vi "3_Speech_Rec_Deploy(file).vi"() -> ()   [LabVIEW 2020]
doc: "This example demonstrates the usage of Deep Learning Toolkit for loading the model pretrained for speech recognition and running for inference."
uses:
  <vilib>/Ngene/Deep Learning Toolkit/Toolkit/NN_Network/Controls/NN_Device.ctl
  <vilib>/Ngene/Deep Learning Toolkit/Toolkit/NN_Network/Controls/NN_Save_Before_Destroy_Options.ctl
  <vilib>/Ngene/Deep Learning Toolkit/Toolkit/NN_Network/API/NN_Set_Input/3D/NN_Set_Input(3D_SGL_idx).vi
  <vilib>/Ngene/Deep Learning Toolkit/Toolkit/Deep_Learning_Toolkit_by_Ngene.lvlib
  <vilib>/vision/NI_Vision_Development_Module.lvlib
panel:
  out "Spectrogram":dbl[][](graph)
  out "Class Labels":string[](array[string])=["dog", "down", "go", "forward", "four", "stop", "backward", "bed", "bird", "learn", "off", "five", "follow", "one", "no", "seven", "on", "cat", "wow", "_background_noise_", "nine", "left", "marvin", "zero", "up", "right", "sheila", "yes", "visual", "six", "two", "house", "eight", "tree", "happy", "three"]
  out "Waveform":waveform(dbl)(graph)={"t0"=timestamp(0 s since 1904-01-01), "dt"=6.25e-05, "Y"=array[16000 elements]}
  out "Class Probabilities":sgl[](array[slide])=[0.99914944, 0.0004657383, 9.833006e-05, 9.4494404e-05, 6.293928e-05, 5.5525186e-05, 1.9071045e-05, 1.3614067e-05, 8.803039e-06, 7.138225e-06, 4.5331067e-06, 4.472217e-06, 3.2921575e-06, 2.4475762e-06, 2.2857214e-06, 2.1201042e-06, 1.2650248e-06, 1.2449445e-06, 1.0311046e-06, 5.384098e-07, 3.8239716e-07, 2.570093e-07, 2.0991196e-07, 1.9032325e-07, 1.7803737e-07, 1.6300649e-07, 1.211693e-07, 9.199508e-08, 4.1726615e-08, 1.04164135e-08, 9.058018e-09, 5.2775126e-09, 2.9758322e-09, 2.9543528e-09, 1.9944413e-09, 8.306618e-10] scale=0.0..1.0
  in  "NN Device":T1=enum."GPU"
  in  "Path to wav":path=path "C:/Users/Nahapet/Downloads/data_speech_commands_v0.02/dog/0ac15fe9_nohash_2.wav"
  in  "Play?":bool=TRUE
  out "Inference Time(sec)":dbl=0.07463920000009239 format="%#_3p"
  in  "Network Configuration File Path":path=path "D:/working/speech_rec/Speech_Rec_net_cfg_26_07_10__17_58_19.cfg"
  in  "Weight File Path":path=path "D:/working/speech_rec/Speech_Rec_weights_26_07_10__17_58_19.bin"
  in  "Stop":bool
  # "Overview: This example demonstrates the use of Deep Learning Toolkit for loading a model pretrained for speech recognition and running it for inference.\nRequirements:\n1. Deep Learning Toolkit for LabVIEW.\n2. NI Vision Development Module.\nInstructions:\nThis example requires the trained model (network topology file .cfg and trained weights file .bin) generated in the previous step.\n1. Provide the trained model files at \"Network Configuration File Path\" and \"Weight File Path\".\n2. Run the VI.\n3. Drag and drop a wav file into the \"Path to wav\" control and observe the prediction results."
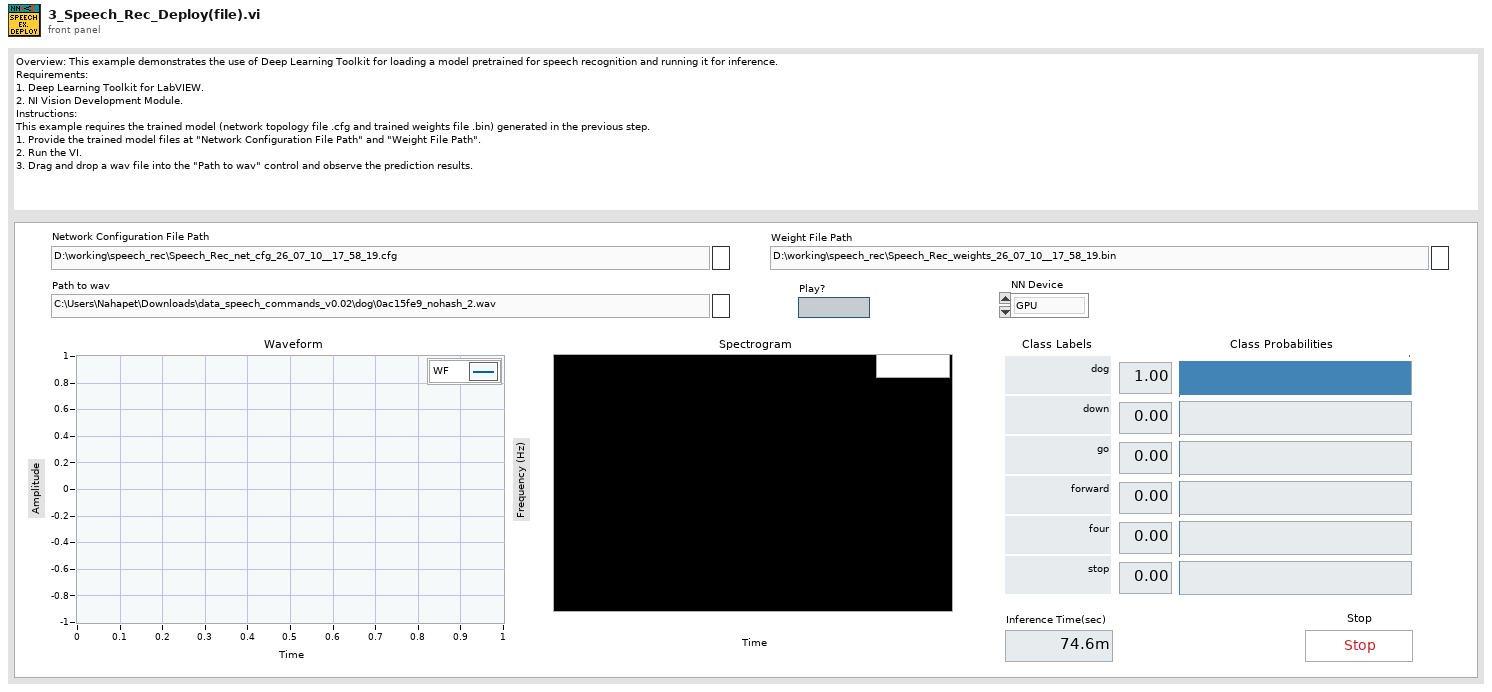
[diagram p1: front panel]
types:
  T1 = typedef "Deep_Learning_Toolkit_by_Ngene.lvlib/NN_Device.ctl" = enum16{"CPU", "GPU"}
  T2 = typedef "Image Type" = u32
  T3 = typedef "Deep_Learning_Toolkit_by_Ngene.lvlib/NN_Save_Before_Destroy_Options.ctl" = cluster{"CFG?":bool, "Weights?":bool, "Render?":bool}
  T4 = typedef "Deep_Learning_Toolkit_by_Ngene.lvlib/NN_Config_Params.ctl" = cluster{"Name":string, "mBatch":i32, "NN_Train_Params":T5, "LR_Decay_Policy":T8, "Labels":string[], "Loss":T10, "Max_WS_Size(B)":i64, "DryRun?":bool}
  T5 = typedef "Deep_Learning_Toolkit_by_Ngene.lvlib/NN_Train_Params.ctl" = cluster{"Optimizer":T6, "Beta_1":sgl, "Beta_2":sgl, "Weight Decay(L1)":sgl, "Weight Decay(L2)":sgl, "Data_Sampling":T7}
  T6 = typedef "Deep_Learning_Toolkit_by_Ngene.lvlib/NN_Train_Optimizer.ctl" = enum16{"SGD", "Adam", "Adagrad", "Adadelta", "RMSProp", "Nesterov"}
  T7 = typedef "Deep_Learning_Toolkit_by_Ngene.lvlib/NN_Train_Data_Sampling.ctl" = enum16{"Random", "Sequential"}
  T8 = typedef "Deep_Learning_Toolkit_by_Ngene.lvlib/NN_LR_Policy_Cfg.ctl" = cluster{"Policy_Type":T9, "LR0":dbl, "k":sgl, "WarmUp_Policy":enum16{"Step", "Ramp"}, "WarmUp_Iter":i32, "WarmUp_Ratio":sgl}
  T9 = typedef "Deep_Learning_Toolkit_by_Ngene.lvlib/NN_LR_Policy_Type.ctl" = enum16{"Manual", "Step", "Exp", "1/t"}
  T10 = typedef "Deep_Learning_Toolkit_by_Ngene.lvlib/NN_Loss_Config_Params.ctl" = cluster{"Loss_Type":T11, "Loss_Conf_Params":variant}
  T11 = typedef "Deep_Learning_Toolkit_by_Ngene.lvlib/NN_Loss_Type.ctl" = enum16{"None", "MSE", "CrossEntropy", "YOLO_v2", "YOLO_v4"}
  T12 = typedef "Deep_Learning_Toolkit_by_Ngene.lvlib/NN_Layer_Config_Params.ctl" = cluster{"Layer_Type":T13, "Layer_Conf_Params":variant, "Input Layers":string[]}
  T13 = typedef "Deep_Learning_Toolkit_by_Ngene.lvlib/NN_Layer_Type.ctl" = enum16{"Input1D", "Input3D", "Conv1D", "Conv2D", "Conv2D_Adv", "MaxPool", "AvgPool", "UpSample", "DropOut3D", "ShortCut", "Concat", "SoftMax3D", "FC", "DropOut", "Softmax", "Flatten", "YOLO_v2", "YOLO_v4", "Activation", "BatchNormalization", "LayerNormalization", "Scale", "Unsupported"}
  T14 = typedef "Deep_Learning_Toolkit_by_Ngene.lvlib/NN.ctl" = cluster{"Name":string, "No of Layers":i32, "mBatch":i32, "Layers":T15[], "Dimty":T16, "Dims_In":T17, "Dims_Out":T17, "Working_Dir":path, "Train?":bool, "Train_Params":T5, "LR_Update_Policy":T8, "Session Data":T18, "Ground_truth":T19, "NNg_hdls":T20, "NN_Device":T1, "GPU Id":i32, "Labels":string[], "Loss_Type":T11, "Loss_Cfg_Prms":variant, "NNG_WS":T21, "DryRun?":bool}
  T15 = typedef "Deep_Learning_Toolkit_by_Ngene.lvlib/NN_Layer_ref.ctl" = refnum<file>
  T16 = typedef "Deep_Learning_Toolkit_by_Ngene.lvlib/NN_In_Out_Dim-ty.ctl" = enum8{"In1D_Out1D", "In3D_Out1D", "In3D_Out3D", "In3D_OutBBox"}
  T17 = typedef "Deep_Learning_Toolkit_by_Ngene.lvlib/NN_Dims(C,H,W).ctl" = cluster{"C":i32, "H":i32, "W":i32}
  T18 = typedef "Deep_Learning_Toolkit_by_Ngene.lvlib/NN_Train_Session_Data.ctl" = cluster{"Epochs":sgl, "Tot_Iter":i32, "LR":sgl, "LR_iter":i32}
  T19 = typedef "Deep_Learning_Toolkit_by_Ngene.lvlib/NN_Ground_truth.ctl" = cluster{"Y":variant}
  T20 = typedef "Deep_Learning_Toolkit_by_Ngene.lvlib/nng_cuda_handles.ctl" = cluster{"cudnn":u64, "cublas":u64, "stream":u64, "curand":u64}
  T21 = typedef "Deep_Learning_Toolkit_by_Ngene.lvlib/NNG_WS.ctl" = cluster{"NNG_WS_Mem":T22, "Max_WS_Size":i64}
  T22 = typedef "Deep_Learning_Toolkit_by_Ngene.lvlib/NNg_WS_Mem_DVR.ctl" = refnum<data-value>
  T23 = typedef "IMAQ Image.ctl" = refnum<image>
  T24 = cluster{"spectral map":dbl[][], "X scale":cluster{"offset":dbl, "multiplier":dbl}, "Y scale":cluster{"offset":dbl, "multiplier":dbl}, "attribute":variant}
  T25 = typedef "Deep_Learning_Toolkit_by_Ngene.lvlib/NN_Layer.ctl" = cluster{"Name":string, "Layer_Data":T26, "Layer_Type":T13, "Dims_In":T17, "Layers_In":T15[], "Dims_Out":T17, "Layers_Out":T15[], "Metrics":T27, "GPU_Data":T28, "mBatch":i32, "NN_Device":T1, "NNg_hdls":T20, "Train?":bool, "Dimty":T29, "RecptField":T30, "Idx":i32}
  T26 = typedef "Deep_Learning_Toolkit_by_Ngene.lvlib/NN_Layer_Data_Refnum.ctl" = refnum<file>
  T27 = typedef "Deep_Learning_Toolkit_by_Ngene.lvlib/NN_Layer_Metrics.ctl" = cluster{"Data":dbl, "Params":dbl, "Ops":dbl}
  T28 = typedef "Deep_Learning_Toolkit_by_Ngene.lvlib/NNg_Layer_Data_Refnum.ctl" = refnum<file>
  T29 = typedef "Deep_Learning_Toolkit_by_Ngene.lvlib/NN_Layer_Dimty.ctl" = enum16{"1D", "3D"}
  T30 = typedef "Deep_Learning_Toolkit_by_Ngene.lvlib/NN_Layer_RF_State.ctl" = cluster{"Dims":T31, "J":T31}
  T31 = typedef "Deep_Learning_Toolkit_by_Ngene.lvlib/NN_Dims(V,H).ctl" = cluster{"V":i32, "H":i32}
  T32 = cluster{"Numeric Control":sgl, "Labels":string}[]
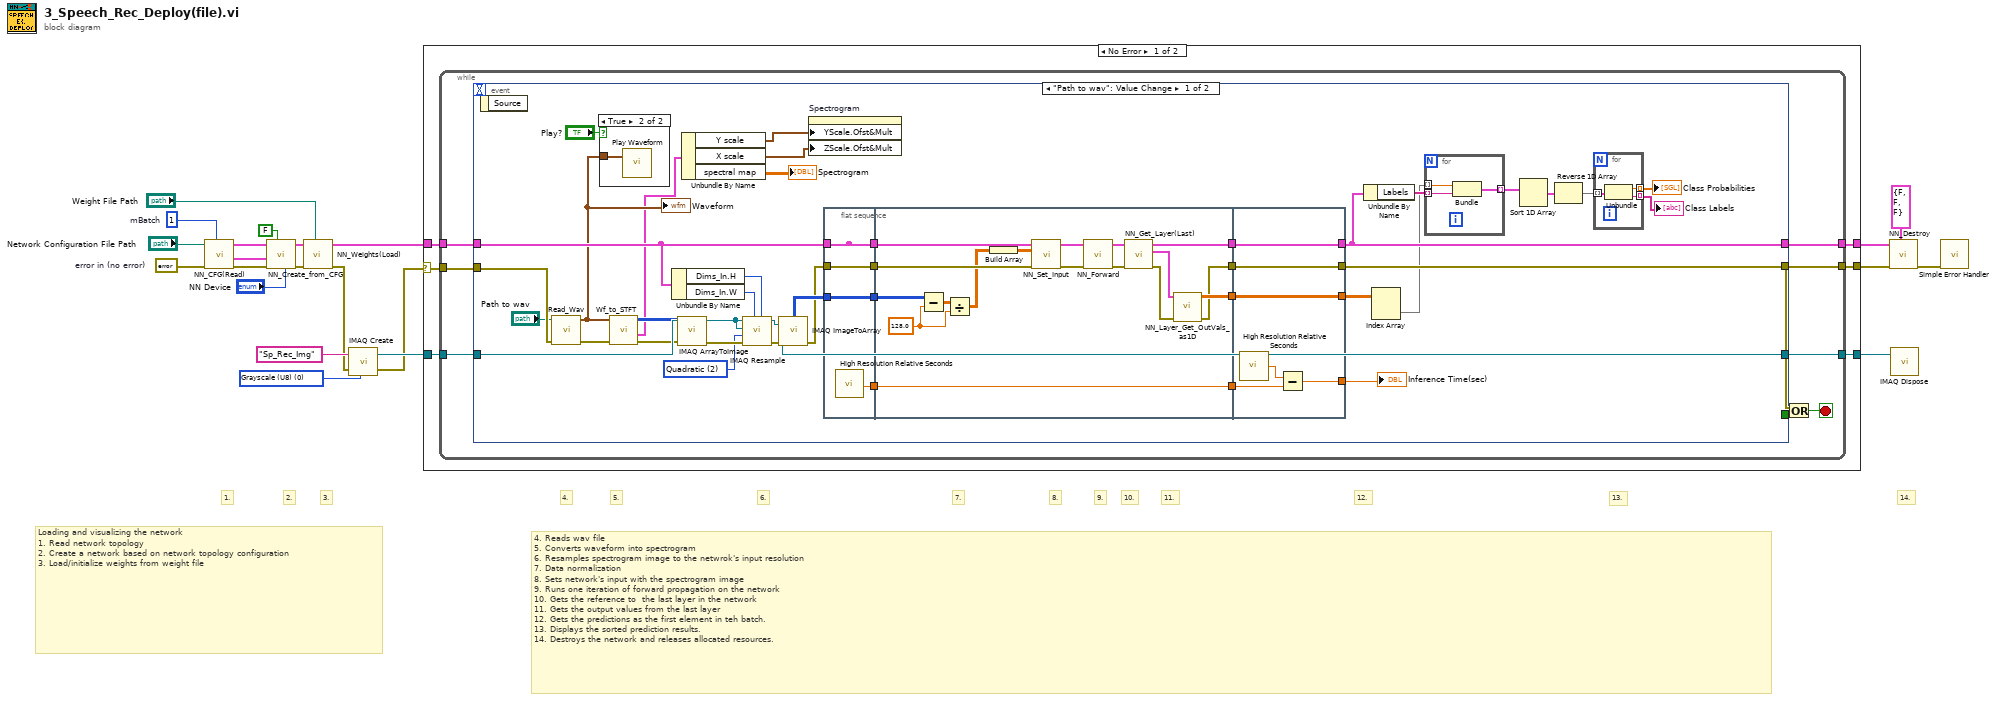
[diagram p0: block diagram]
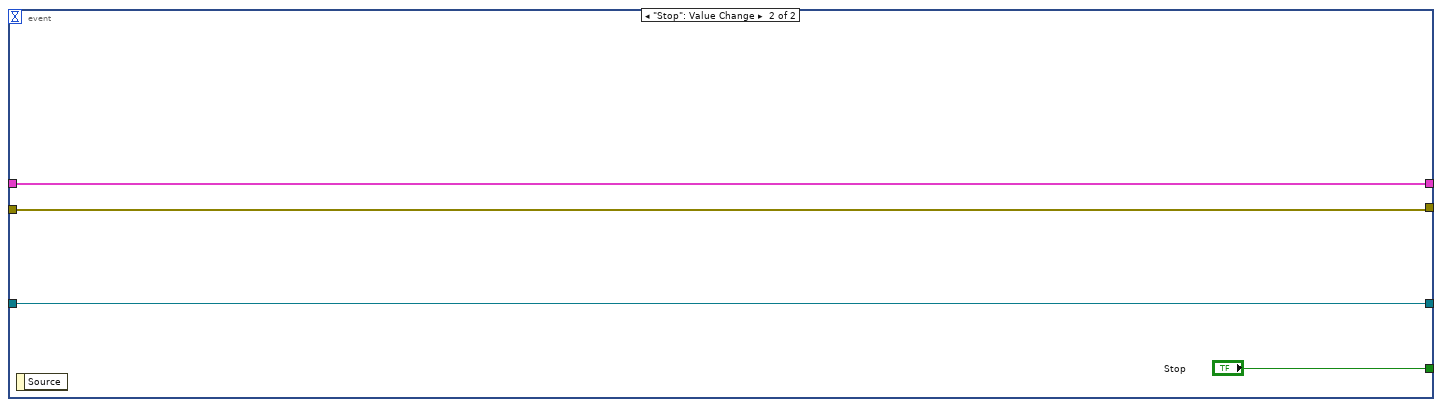
[diagram p3: hidden frame]
diagram:
  w2 = 1  # mBatch
  w14 = errorcluster {"status"=FALSE, "code"=0, "source"=""}  # error in (no error)
  w18 = T2 0 items=["Grayscale (U8)", "Grayscale (I16)", "Grayscale (SGL)", "Complex (CSG)", "RGB (U32)", "HSL (U32)", "RGB (U64)", "Grayscale (U16)"] ("Image Type")
  # "13."
  # "14."
  # "12."
  # "11."
  # "10."
  # "9."
  # "4. Reads wav file\n5. Converts waveform into spectrogram\n6. Resamples spectrogram image to the netwrok's input resolution\n7. Data normalization\n8. Sets network's input with the spectrogram image\n9. Runs one iteration of forward propagation on the network\n10. Gets the reference to  the last layer in the network\n11. Gets the output values from the last layer\n12. Gets the predictions as the first element in teh batch.\n13. Displays the sorted prediction results.\n14. Destroys the network and releases allocated resources."
  # "8."
  # "7."
  # "6."
  # "5."
  # "4."
  # "Loading and visualizing the network\n1. Read network topology\n2. Create a network based on network topology configuration\n3. Load/initialize weights from weight file"
  # "3."
  # "2."
  # "1."
  n1 = call <vilib>:"NN_CFG(Read).vi"("mBatch"=w2, "error in (no error)"=w14, "CFG file path"="Network Configuration File Path") -> ("error out"=w16:errorcluster, "Net_Cfg"=w15:T4, "Layer_Cfg"=w6:T12[])  [unwired: 6 in]
  n2 = call <vilib>:"NN_Create_from_CFG.vi"("NN_Device"="NN Device", "Train? (false)"=FALSE, "error in (no error)"=w16, "Net_Cfg"=w15, "Layer_Cfg"=w6) -> ("error out"=w12:errorcluster, "NN out"=w7:T14)  [unwired: 5 in]
  n3 = call <vilib>:"NN_Weights(Load).vi"("Weight File Path"="Weight File Path", "error in (no error)"=w12, "NN in"=w7) -> ("error out"=w4:errorcluster, "NN out"=w10:T14)  [unwired: 7 in]
  n4 = call "IMAQ Create"("Image Name"="Sp_Rec_Img", "Image Type"=w18, "error in (no error)"=w4) -> ("New Image"=w17:T23, "error out"=w3:errorcluster)  [unwired: 2 in]
  n5 = case shown="No Error" w3 {
    selector: w3 -> [w27 w118]
    tunnel: w10 -> [w24 w117]
    tunnel: [w28 w117] -> w20
    tunnel: [w26 w118] -> w8
    tunnel: w17 -> [w25 w116]
    tunnel: [w23 w116] -> w9
    frame No Error {
      n6 = while {
        tunnel: w27 -> [w35]
        tunnel: [w32] -> w28
        tunnel: [w30] -> w26
        tunnel: w25 -> [w34]
        tunnel: w24 -> [w33]
        tunnel: [w29] -> w23
        stop <- w36 stop-if-true
        n7 = event shown="[0] \"Path to wav\": Value Change" {
          selector: _ -> [_ _]
          dyn-events: _ -> [_ _]
          timeout: _ -> [_ _]
          tunnel: [_ "Stop"] -> w31
          tunnel: [w47 w112] -> w32
          tunnel: w35 -> [w72 w115]
          tunnel: [w52 w114] -> w29
          tunnel: w34 -> [w74 w114]
          tunnel: [w54 w115] -> w30
          tunnel: w33 -> [w51 w112]
          event "Path to wav": Value Change {
            w48 = u32 2 items=["Zero Order", "Bi-Linear", "Quadratic", "Cubic Spline"] ("Interpolation Type")
            n8 = event-data() -> ()  [unwired: 1 in, 1 out]
            n9 = call "Read_Wav.vi"("error in (no error)"=w72, "Path to wav"="Path to wav") -> ("error out"=w73:errorcluster, "wf"=w44:waveform(dbl))  [unwired: 8 in]
            "Waveform" <- w44
            n10 = case shown="True" "Play?" {
              tunnel: w44 -> [_ w111]
              frame False {
              }
              frame True {
                n11 = call "Play Waveform"("Data"=w111) -> ()  [unwired: 18 in, 1 out]
              }
            }
            n12 = call "Wf_to_STFT.vi"("error in (no error)"=w73, "WF"=w44) -> ("error out"=w69:errorcluster, "STFT"=w43:T24, "Image_data"=w70:u8[][])  [unwired: 7 in]
            n13 = Unbundle By Name(w51) -> ("Dims_In.H"=w50:i32, "Dims_In.W"=w49:i32)
            n14 = call "IMAQ ArrayToImage"("error in (no error)"=w69, "Image Pixels (U8)"=w70, "Image"=w74) -> ("error out"=w76:errorcluster, "Image Out"=w77:T23)  [unwired: 7 in]
            n15 = Unbundle By Name(w43) -> ("Y scale"=w38:cluster{"offset":dbl, "multiplier":dbl}, "X scale"=w37:cluster{"offset":dbl, "multiplier":dbl}, "spectral map"=→"Spectrogram":dbl[][])
            n16 = call "IMAQ Resample"("X Resolution"=w50, "Y Resolution"=w49, "error in (no error)"=w76, "Interpolation Type"=w48, "Image Dst"=w77, "Image Src"=w77) -> ("error out"=w75:errorcluster, "Image Dst Out"=w52:T23)  [unwired: 4 in]
            n17 = call "IMAQ ImageToArray"("error in (no error)"=w75, "Image"=w52) -> ("error out"=w55:errorcluster, "Image Pixels (U8)"=w56:u8[][])  [unwired: 2 in, 3 out]
            n18 = property on="Spectrogram" class="IntGraph (strict)"("YScale.Ofst&Mult"=w38, "ZScale.Ofst&Mult"=w37) -> ()  [unwired: 2 in, 2 out]
            n19 = flat-sequence {
              tunnel: w55 -> [w84]
              tunnel: [w81] -> _
              tunnel: [w81] -> w67
              tunnel: [w84] -> w66
              tunnel: [w83] -> w65
              tunnel: w56 -> [w82]
              tunnel: [w82] -> w64
              tunnel: w51 -> [w81]
              tunnel: w67 -> [w97]
              tunnel: w66 -> [w100]
              tunnel: [w101] -> w63
              tunnel: [w99] -> w62
              tunnel: w65 -> [w96]
              tunnel: [w96] -> w61
              tunnel: [w98] -> w60
              tunnel: w64 -> [w86]
              tunnel: [w106] -> w47
              tunnel: [w107] -> w59
              tunnel: w63 -> [w107]
              tunnel: w62 -> [w106]
              tunnel: w61 -> [w105]
              tunnel: w60 -> [w103]
              tunnel: [w103] -> w54
              tunnel: [w102] -> w53
              frame #0 {
                n20 = call <vilib>:"High Resolution Relative Seconds.vi"() -> ("relative seconds"=w83:dbl)
              }
              frame #1 {
                w87 = sgl 128.0 ("dimension size")
                n21 = Subtract(x=w86, y=w87) -> (x-y=w90:sgl[][])
                n22 = Divide(x=w90, y=w87) -> (x/y=w89:sgl[][])
                n23 = Build Array(w89) -> (w85:sgl[][][])
                n24 = call-poly <vilib>:"NN_Set_Input.vi"("error in (no error)"=w100, "Data_In(3D_SGL)"=w85, "NN in"=w97) -> ("error out"=w88:errorcluster, "NN out"=w93:T14)  [unwired: 7 in]
                n25 = call <vilib>:"NN_Forward.vi"("error in (no error)"=w88, "NN in"=w93) -> ("error out"=w92:errorcluster, "NN out"=w91:T14)  [unwired: 6 in, 2 out]
                n26 = call <vilib>:"NN_Get_Layer(Last).vi"("error in (no error)"=w92, "NN in"=w91) -> ("error out"=w95:errorcluster, "Last_Layer"=w94:T25, "NN out"=w99:T14)  [unwired: 6 in, 1 out]
                n27 = call <vilib>:"NN_Layer_Get_OutVals_as1D.vi"("error in (no error)"=w95, "Layer"=w94) -> ("error out"=w98:errorcluster, "Out(as1D)"=w101:sgl[][])  [unwired: 8 in]
              }
              frame #2 {
                n28 = call <vilib>:"High Resolution Relative Seconds.vi"() -> ("relative seconds"=w104:dbl)
                n29 = Subtract(x=w104, y=w105) -> (x-y=w102:dbl)
              }
            }
            n30 = Unbundle By Name(w47) -> ("Labels"=w46:string[])
            n31 = Index Array(array=w59) -> (element=w45:sgl[])  [unwired: 2 in]
            n32 = for {
              tunnel: w45 -> [w110] mode=indexing
              tunnel: w46 -> [w109] mode=indexing
              tunnel: [w108] -> w58 mode=indexing
              n33 = Bundle("Numeric Control"=w110, "Labels"=w109) -> (w108:cluster{"Numeric Control":sgl, "Labels":string})  [unwired: 1 in]
            }
            n34 = Sort 1D Array(array=w58) -> (sorted array=w57:T32)
            n35 = Reverse 1D Array(array=w57) -> (reversed array=w41:T32)
            n36 = for {
              tunnel: w41 -> [w80] mode=indexing
              tunnel: [w79] -> w39 mode=indexing
              tunnel: [w78] -> w40 mode=indexing
              n37 = Unbundle(w80) -> ("Numeric Control"=w79:sgl, "Labels"=w78:string)
            }
            "Class Labels" <- w40
            "Class Probabilities" <- w39
            "Inference Time(sec)" <- w53
          }
          event "Stop": Value Change {
            # "Stop the VI."
            n38 = event-data() -> ()  [unwired: 1 in, 1 out]
          }
        }
        n39 = Or(x=w30, y=w31) -> (x .or. y?=w36:bool)
      }
    }
    frame Error {
    }
  }
  n40 = call <vilib>:"NN_Destroy.vi"("Save (T, T, T)"=T3 {"CFG?"=FALSE, "Weights?"=FALSE, "Render?"=FALSE} ("Save_Config"), "error in (no error)"=w8, "NN in"=w20) -> ("error out"=w22:errorcluster)  [unwired: 7 in, 1 out]
  n41 = call "IMAQ Dispose"("Image"=w9) -> ()  [unwired: 5 in, 1 out]
  n42 = call <vilib>:"Simple Error Handler.vi"("error in (no error)"=w22) -> ()  [unwired: 4 in, 5 out]
